vi "CPP_BandLimitBoost.vi"(4 "CutoffIndex":dbl, 5 "AmplitudeBoost":dbl[](array[numeric])) -> (2 "BandLimitedBoost":dbl[](array[numeric]))   [LabVIEW 2012]
uses:
  <vilib>/Analysis/NI_AALBase.lvlib
panel:
  in  "Combo Box":string(combo)="Cosine"
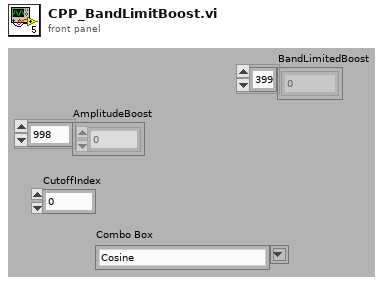
[diagram p1: front panel]
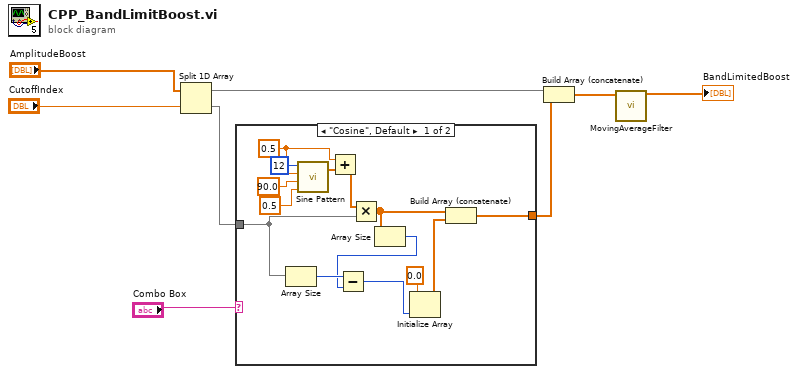
[diagram p0: block diagram]
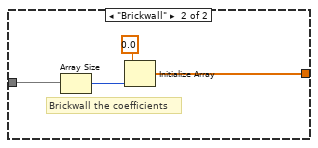
[diagram p2: hidden frame]
diagram:
  n1 = Split 1D Array(array="AmplitudeBoost", index="CutoffIndex") -> (first subarray=w6:dbl[], second subarray=w7:dbl[])
  n2 = case shown="\"Cosine\", Default" "Combo Box" {
    tunnel: [w15 w26] -> w8
    tunnel: w7 -> [w17 w24]
    frame "Cosine", Default {
      w18 = 0.5 ("amplitude")
      n3 = Array Size(array=w17) -> (size(s)=w13:i32)
      n4 = call <vilib>:"Sine Pattern.vi"("cycles"=0.5, "phase(degrees)"=90.0, "amplitude"=w18, "samples"=12) -> ("Sinusoidal Pattern"=w21:dbl[])  [unwired: 1 out]
      n5 = Add(x=w18, y=w21) -> (x+y=w20:dbl[])
      n6 = Multiply(x=w20, y=w17) -> (x*y=w14:dbl[])
      n7 = Array Size(array=w14) -> (size(s)=w12:i32)
      n8 = Subtract(x=w13, y=w12) -> (x-y=w11:i32)
      n9 = Initialize Array(0.0 ("element"), w11) -> (w10:dbl[])
      n10 = Build Array (concatenate)(w14, w10) -> (w15:dbl[])
    }
    frame "Brickwall" {
      # "Brickwall the coefficients"
      n11 = Array Size(array=w24) -> (size(s)=w25:i32)
      n12 = Initialize Array(0.0 ("element"), w25) -> (w26:dbl[])
    }
  }
  n13 = Build Array (concatenate)(w6, w8) -> (w2:dbl[])
  n14 = call "MovingAverageFilter.vi"("X"=w2) -> ("Filtered X"=→"BandLimitedBoost":dbl[])  [unwired: 10 in]
